vi "apply sensor geometry.vi"(10 "Posture In":dbl[](array[numeric]), 11 "IF readings\n(meters)":dbl[](array[numeric]) format="%_6g") -> (2 "ir distances rf":dbl[][](array[numeric]), 3 "ir distances wf":dbl[][](array[numeric]))   [LabVIEW 2016]
uses:
  <vilib>/Analysis/coordinate.llb/2D Cartesian Coordinate Rotation (Scalar).vi
  <vilib>/Analysis/coordinate.llb/2D Cartesian Coordinate Rotation (Array).vi
  <vilib>/Analysis/NI_AALPro.lvlib
panel:
  in  "Sensor placement":dbl[][](array[numeric])=[[-0.12, -0.055, 0.0, 0.055, 0.12], [0.0, 0.163, 0.179, 0.163, 0.0], [3.1415, 2.356, 1.571, 0.7853, 0.0]]
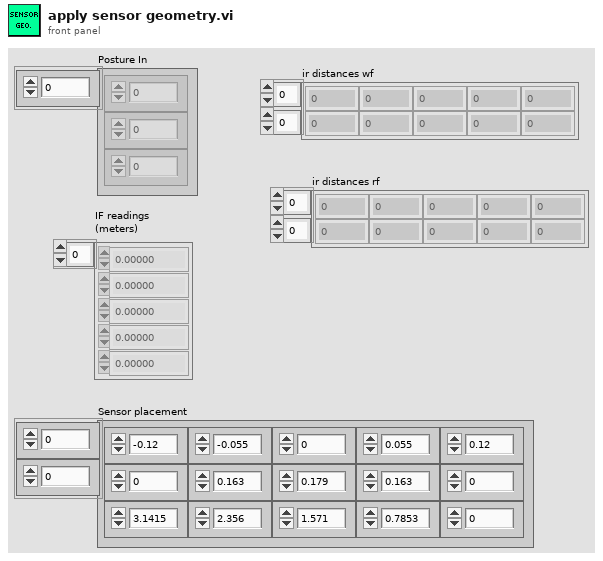
[diagram p1: front panel]
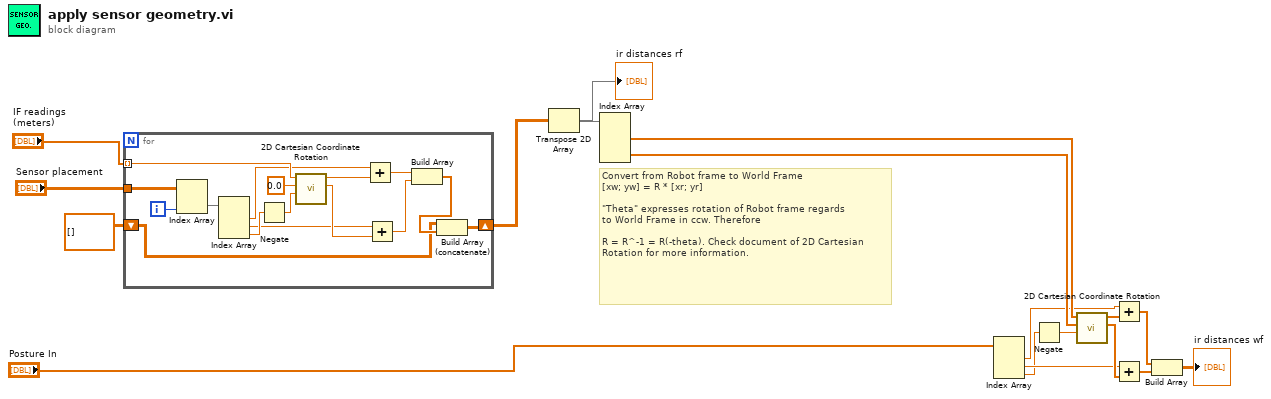
[diagram p0: block diagram]
diagram:
  # "Convert from Robot frame to World Frame\n[xw; yw] = R * [xr; yr]\n\n\"Theta\" expresses rotation of Robot frame regards \nto World Frame in ccw. Therefore\n\nR = R^-1 = R(-theta). Check document of 2D Cartesian\nRotation for more information."
  n1 = for {
    tunnel: "IF readings\n(meters)" -> [w30] mode=indexing
    tunnel: "Sensor placement" -> [w33]
    shift-right: [w18] -> w2
    shift-left: dbl[][] [] -> [w19]
    i -> [w32]
    n2 = Index Array(array=w33, index (col)=w32) -> (element=w31:dbl[])  [unwired: 1 in]
    n3 = Index Array(array=w31) -> (element #1=w25:dbl, element #2=w23:dbl, element #3=w28:dbl)  [unwired: 3 in]
    n4 = Negate(x=w28) -> (-x=w27:dbl)
    n5 = call-poly <vilib>:"2D Cartesian Coordinate Rotation.vi"("theta"=w27, "y"=0.0, "x"=w30) -> ("y out"=w24:dbl, "x out"=w26:dbl)  [unwired: 6 in, 1 out]
    n6 = Add(x=w25, y=w26) -> (x+y=w22:dbl)
    n7 = Add(x=w23, y=w24) -> (x+y=w21:dbl)
    n8 = Build Array(w22, w21) -> (w20:dbl[])
    n9 = Build Array (concatenate)(w19, w20) -> (w18:dbl[][])
  }
  n10 = Transpose 2D Array(2D array=w2) -> (transposed array=w1:dbl[][])
  "ir distances rf" <- w1
  n11 = Index Array(array=w1) -> (element #1=w17:dbl[], element #2=w16:dbl[])  [unwired: 4 in]
  n12 = Index Array(array="Posture In") -> (element #1=w8:dbl, element #2=w7:dbl, element #3=w6:dbl)  [unwired: 3 in]
  n13 = Negate(x=w6) -> (-x=w10:dbl)
  n14 = call-poly <vilib>:"2D Cartesian Coordinate Rotation.vi"("theta"=w10, "Y"=w16, "X"=w17) -> ("Y Out"=w14:dbl[], "X Out"=w15:dbl[])  [unwired: 6 in, 1 out]
  n15 = Add(x=w8, y=w15) -> (x+y=w13:dbl[])
  n16 = Add(x=w7, y=w14) -> (x+y=w12:dbl[])
  n17 = Build Array(w13, w12) -> (→"ir distances wf":dbl[][])
